vi "Advance Loop Get Images.vi"() -> ()   [LabVIEW 2017]
uses:
  IMAQCV/PIIO/Core/PIIO DIO.ctl
  IMAQCV/IMAQCV.lvlib
  IMAQCV/PIIO.lvlib
panel:
  in  "PIN":T1 items=["L1", "L2"]
  in  "Start Pixel Index":u16
  in  "Number of LEDs":u16=40
  in  "Green":u8(slide) scale=0.0..255.0
  in  "Blue":u8(slide) scale=0.0..255.0
  out "LED Color":u32(colorbox)
  in  "Red":u8(slide) scale=0.0..255.0
  in  "Shutter (us, 0=auto)":i32
  in  "Effect":T2(ring)
  in  "Meter":enum16{"AVERAGE", "SPOT", "BACKLIT", "MATRIX"}(ring)
  in  "AWB":T3(ring)
  in  "Flip Vertical":bool
  in  "Flip Horizontal":bool
  in  "Rotation":u16(ring) items=["0", "90", "180", "270"]
  in  "Sharpness":i32(slide)=50 scale=0.0..100.0
  in  "Saturation":i32(slide)=50 scale=0.0..100.0
  in  "Contrast":i32(slide)=50 scale=0.0..100.0
  in  "Brightness":i32(slide)=50 scale=0.0..100.0
  in  "Gain (0=auto)":i32(slide) scale=0.0..100.0
  in  "FPS":i32=30
  in  "Type":enum16{"GRAY", "COLOR"}(ring)
  out "picture":picture
  in  "Image Size":T4(ring)
  in  "Image Index":u32
  in  "stop":bool
  in  "Save Image":bool
  in  "Image File Path":path=path "c:/vision/project-01/camera-000.jpg"
  out "Loop Rate (Hz)":u32
  # "Raspberry Pi Camera"
  # "WS2812 RGB LED"
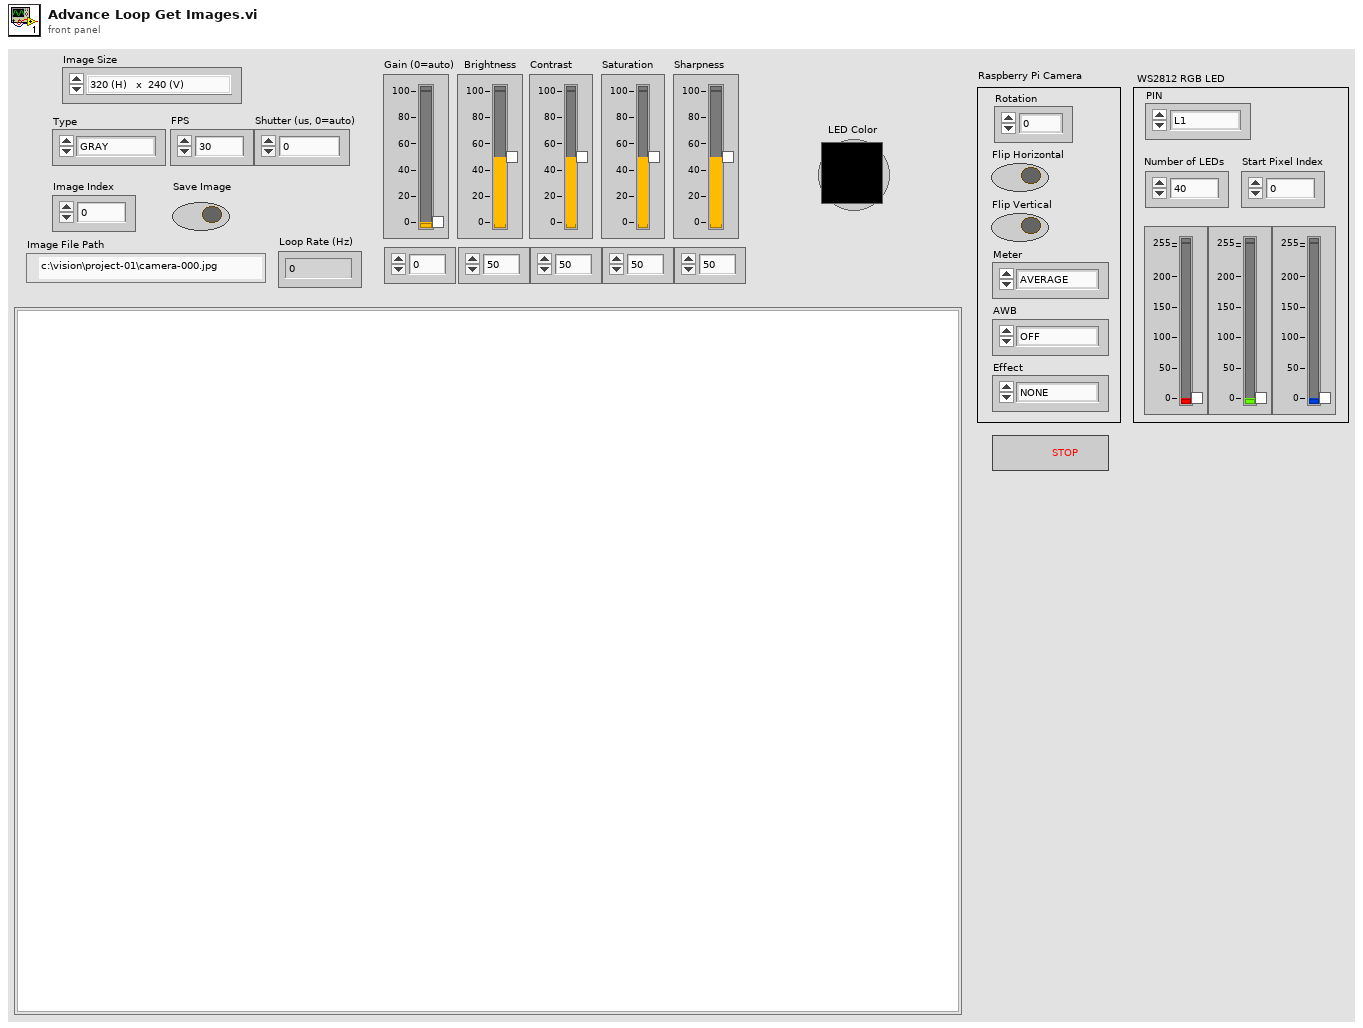
[diagram p1: front panel]
types:
  T1 = typedef "PIIO.lvlib/PIIO DIO.ctl" = u8
  T2 = enum16{"NONE", "NEGATIVE", "SOLARIZE", "SKETCH", "DENOISE", "EMBOSS", "OILPAINT", "HATCH", "GPEN", "PASTEL", "WATERCOLOR", "FILM", "BLUR", "SATURATION", "COLORSWAP", "WASHEDOUT", "POSTERISE", "COLORPOINT", "COLORBALANCE", "CARTOON"}
  T3 = enum16{"OFF", "AUTO", "SUNLIGHT", "CLOUDY", "SHADE", "TUNGSTEN", "FLUORESCENT", "INCANDESCENT", "FLASH"}
  T4 = enum16{"320 (H)   x  240 (V)", "352(H)    x  288 (V)", "640 (H)   x  480 (V) ", "800 (H)   x  600 (V)", "1024 (H) x  768 (V)", "1280 (H) x  720 (V)", "1280 (H) x  960 (V)", "1280 (H) x 1024 (V)", "1920 (H) x 1080 (V)"}
  T5 = typedef "Image Type" = u32
  T6 = typedef "IMAQCV.lvlib/IMAQCV Image.ctl" = refnum<vi>
  T7 = typedef "IMAQ Image.ctl" = refnum<image>
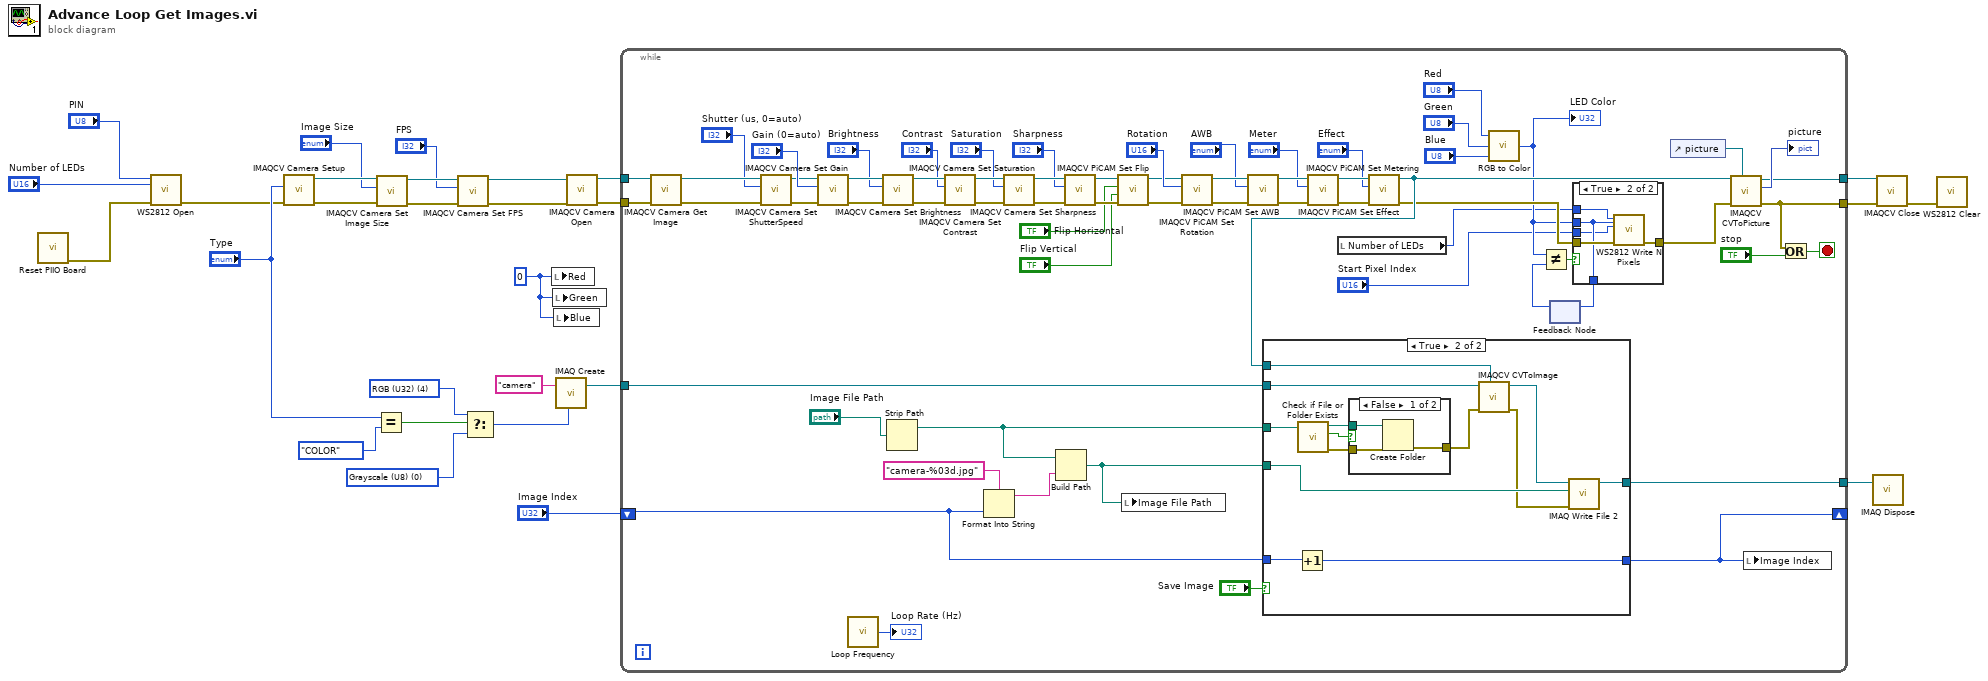
[diagram p0: block diagram]
diagram:
  w2 = u8 0 ("Red")
  w14 = T5 0 items=["Grayscale (U8)", "Grayscale (I16)", "Grayscale (SGL)", "Complex (CSG)", "RGB (U32)", "HSL (U32)", "RGB (U64)", "Grayscale (U16)"] ("Image Type")
  w13 = T5 4 items=["Grayscale (U8)", "Grayscale (I16)", "Grayscale (SGL)", "Complex (CSG)", "RGB (U32)", "HSL (U32)", "RGB (U64)", "Grayscale (U16)"] ("Image Type")
  n1 = call "Reset PIIO Board.vi"() -> ("error out"=w6:errorcluster)  [unwired: 11 in]
  n2 = call "WS2812 Open.vi"("Error In"=w6, "Number of LEDs"="Number of LEDs", "PIN"="PIN") -> ("Error Out"=w5:errorcluster)  [unwired: 8 in]
  n3 = call "IMAQCV Camera Setup.vi"("error in (no error)"=w5, "type"="Type") -> ("error out"=w26:errorcluster, "image out"=w25:T6)  [unwired: 8 in]
  n4 = Equal?(x="Type", y=enum16{"GRAY", "COLOR"}."COLOR" ("type")) -> (x = y?=w15:bool)
  n5 = call "IMAQCV Camera Set Image Size.vi"("error in (no error)"=w26, "Image Size"="Image Size", "image in"=w25) -> ("error out"=w11:errorcluster, "image out"=w10:T6)  [unwired: 7 in]
  n6 = call "IMAQCV Camera Set FPS.vi"("error in (no error)"=w11, "FPS"="FPS", "image in"=w10) -> ("error out"=w8:errorcluster, "image out"=w9:T6)  [unwired: 7 in]
  n7 = Select(t=w13, s=w15, f=w14) -> (s? t:f=w12:T5)
  n8 = local write "Red"(w2) -> ()
  n9 = local write "Green"(w2) -> ()
  n10 = local write "Blue"(w2) -> ()
  n11 = call "IMAQ Create"("Image Name"="camera", "Image Type"=w12) -> ("New Image"=w20:T7)  [unwired: 2 in, 2 out]
  n12 = call "IMAQCV Camera Open.vi"("error in (no error)"=w8, "image in"=w9) -> ("error out"=w24:errorcluster, "image out"=w23:T6)  [unwired: 8 in]
  n13 = while {
    tunnel: w23 -> [w82]
    tunnel: [w77] -> w21
    shift-right: [w84] -> _
    shift-left: "Image Index" -> [w85]
    tunnel: w24 -> [w83]
    tunnel: w20 -> [w80]
    tunnel: [w79] -> w19
    tunnel: [w76] -> w18
    stop <- w92 stop-if-true
    n14 = call "IMAQCV Camera Get Image.vi"("error in (no error)"=w83, "image in"=w82) -> ("error out"=w44:errorcluster, "image out"=w43:T6)  [unwired: 8 in]
    n15 = call "IMAQCV Camera Set ShutterSpeed.vi"("error in (no error)"=w44, "shutter speed (us, 0=auto)"="Shutter (us, 0=auto)", "image in"=w43) -> ("error out"=w45:errorcluster, "image out"=w42:T6)  [unwired: 7 in]
    n16 = call "IMAQCV Camera Set Gain.vi"("error in (no error)"=w45, "gain (0=auto)"="Gain (0=auto)", "image in"=w42) -> ("error out"=w74:errorcluster, "image out"=w75:T6)  [unwired: 7 in]
    n17 = call "Loop Frequency.vi"() -> ("Loop Rate (Hz)"=→"Loop Rate (Hz)":u32)  [unwired: 1 out]
    n18 = call "IMAQCV Camera Set Brightness.vi"("error in (no error)"=w74, "brightness"="Brightness", "image in"=w75) -> ("error out"=w73:errorcluster, "image out"=w70:T6)  [unwired: 7 in]
    n19 = Strip Path(path="Image File Path") -> (stripped path=w86:path)  [unwired: 1 out]
    n20 = call "IMAQCV Camera Set Contrast.vi"("error in (no error)"=w73, "contrast"="Contrast", "image in"=w70) -> ("error out"=w72:errorcluster, "image out"=w69:T6)  [unwired: 7 in]
    n21 = Format Into String(format string="camera-%03d.jpg", w85) -> (resulting string=w88:string)  [unwired: 2 in, 1 out]
    n22 = call "IMAQCV Camera Set Saturation.vi"("error in (no error)"=w72, "saturation"="Saturation", "image in"=w69) -> ("error out"=w71:errorcluster, "image out"=w68:T6)  [unwired: 7 in]
    n23 = Build Path(base path=w86, name or relative path=w88) -> (appended path=w87:path)
    n24 = call "IMAQCV Camera Set Sharpness.vi"("error in (no error)"=w71, "sharpness"="Sharpness", "image in"=w68) -> ("error out"=w61:errorcluster, "image out"=w60:T6)  [unwired: 7 in]
    n25 = call "IMAQCV PiCAM Set Flip.vi"("error in (no error)"=w61, "vertical"="Flip Vertical", "horizontal"="Flip Horizontal", "image in"=w60) -> ("error out"=w59:errorcluster, "image out"=w58:T6)  [unwired: 6 in]
    n26 = local write "Image File Path"(w87) -> ()
    n27 = call "IMAQCV PiCAM Set Rotation.vi"("error in (no error)"=w59, "Rotation"="Rotation", "image in"=w58) -> ("error out"=w55:errorcluster, "image out"=w54:T6)  [unwired: 7 in]
    n28 = call "IMAQCV PiCAM Set AWB.vi"("error in (no error)"=w55, "AWB"="AWB", "image in"=w54) -> ("error out"=w52:errorcluster, "image out"=w50:T6)  [unwired: 7 in]
    n29 = call "IMAQCV PiCAM Set Metering.vi"("error in (no error)"=w52, "mode"="Meter", "image in"=w50) -> ("error out"=w51:errorcluster, "image out"=w49:T6)  [unwired: 7 in]
    n30 = local read "Number of LEDs"() -> (w30:u16)
    n31 = call "IMAQCV PiCAM Set Effect.vi"("error in (no error)"=w51, "effect"="Effect", "image in"=w49) -> ("error out"=w39:errorcluster, "image out"=w48:T6)  [unwired: 7 in]
    n32 = case shown="True" "Save Image" {
      tunnel: w87 -> [_ w111]
      tunnel: w86 -> [_ w115]
      tunnel: w85 -> [w102 w110]
      tunnel: [w102 w109] -> w84
      tunnel: w80 -> [w101 w105]
      tunnel: [w101 w104] -> w79
      tunnel: w48 -> [_ w103]
      frame False {
      }
      frame True {
        n33 = Increment(x=w110) -> (x+1=w109:u32)
        n34 = call <vilib>:"Check if File or Folder Exists.vi"("path"=w115) -> ("error out"=w112:errorcluster, "file or folder exists?"=w114:bool, "dup path"=w113:path)  [unwired: 8 in]
        n35 = case shown="False" w114 {
          tunnel: w113 -> [w118 _]
          tunnel: w112 -> [w117 w119]
          tunnel: [w116 w119] -> w107
          frame False {
            n36 = Create Folder(path (use dialog)=w118, error in=w117) -> (error out=w116:errorcluster)  [unwired: 1 in, 2 out]
          }
          frame True {
          }
        }
        n37 = call "IMAQCV CVToImage.vi"("cvimage in"=w103, "error in (no error)"=w107, "Variant In"=w105) -> ("error out"=w106:errorcluster, "Variant Out"=w108:refnum<image>)  [unwired: 7 in]
        n38 = call-poly "IMAQ Write File 2"("error in (no error)"=w106, "File Path"=w111, "Image"=w108) -> ("Image Out (duplicate)"=w104:T7)  [unwired: 7 in, 1 out]
      }
    }
    n39 = call <vilib>:"RGB to Color.vi"("B"="Blue", "G"="Green", "R"="Red") -> ("Color"=w33:u32)
    "LED Color" <- w33
    n40 = feedback #1() -> (w31:u32)  [unwired: 1 in]
    n41 = Not Equal?(x=w33, y=w31) -> (x != y?=w34:bool)
    n42 = case shown="True" w34 {
      tunnel: w39 -> [w95 w100]
      tunnel: [w95 w99] -> w38
      tunnel: w33 -> [w94 w98]
      tunnel: [w94 w98] -> w32
      tunnel: w30 -> [_ w97]
      tunnel: "Start Pixel Index" -> [_ w96]
      frame False {
      }
      frame True {
        n43 = call "WS2812 Write N Pixels.vi"("LED Color"=w98, "Error In"=w100, "Start Pixel Index"=w96, "Number of LEDs"=w97) -> ("Error Out"=w99:errorcluster)  [unwired: 7 in]
      }
    }
    n44 = feedback-in #1(w32) -> ()
    n45 = control-ref of="picture"() -> (w40:refnum<vi>)
    n46 = call "IMAQCV CVToPicture.vi"("picture ref"=w40, "error in (no error)"=w38, "image"=w48) -> ("error out"=w76:errorcluster, "picture"=→"picture":picture, "image out"=w77:T6)  [unwired: 6 in]
    n47 = local write "Image Index"(w84) -> ()
    n48 = Or(x=w76, y="stop") -> (x .or. y?=w92:bool)
  }
  n49 = call "IMAQ Dispose"("Image"=w19) -> ()  [unwired: 5 in, 1 out]
  n50 = call "IMAQCV Close.vi"("error in (no error)"=w18, "Image"=w21) -> ("error out"=w4:errorcluster)  [unwired: 9 in]
  n51 = call "WS2812 Clear.vi"("Error In"=w4) -> ()  [unwired: 10 in, 1 out]
